vi "Single Tone Audio Measurements (N Ch).vi"(6 "units settings":T2, 8 "error in":errorcluster, 10 "measurement settings":T5={"Band start"=20.0, "Band stop"=20000.0, "Amplitude"=1.0, "Frequency"=1000.0, "Full scale range"=3.16}, 11 "waveforms":waveform(dbl)[](array[waveform])) -> (0 "error out":errorcluster, 1 "spectra":cluster{"x0":dbl, "dx":dbl, "magnitude":dbl[]}[](array[cluster]), 2 "waveforms":waveform(dbl)[](array[waveform]), 3 "results":T1[](array[typedef]))   [LabVIEW 2021]
uses:
  controls/single tone audio measurement settings.ctl
  controls/units settings.ctl
  controls/units - snr.ctl
  controls/units - ratio.ctl
  controls/single tone audio measurements.ctl
  <vilib>/addons/_NISVFA/_Shared subVIs/Common/SVL Set dB Reference (N Ch - 1 Ref).vi
  <vilib>/addons/Sound and Vibration/svt_Single Tone Measurements/SVT Spurious Free Dynamic Range (Frequency) (1 Ch).vi
  <vilib>/addons/_NISVFA/_Spectrum Processing/SVFA Unit Conversion (Complex) (1 Ch).vi
  <vilib>/addons/_NISVFA/_Shared subVIs/Common/SVL Set dB Reference (1 Ch).vi
  <vilib>/addons/_NISVFA/_Spectrum Processing/SVFA Get Spectrum Subset.vi
  <vilib>/addons/_NISVFA/_Spectrum Processing/SVFA Get Spectrum Subset (Complex) (1 Ch).vi
  <vilib>/addons/_NISVFA/_Shared subVIs/Common/svc_Window Parameters.vi
  <vilib>/addons/_NISVFA/_Shared subVIs/Common/svc_Extract Single Tone Information (complex).vi
  <vilib>/addons/_NISVFA/_Shared subVIs/Common/svc_Check Frequency Range in Spectrum.vi
  <vilib>/addons/_NISVFA/_Spectrum Processing/SVFA Spectrum Peak Search.vi
  <vilib>/addons/_NISVFA/_Spectrum Processing/SVFA Spectrum Peak Search (1 Ch).vi
  <vilib>/addons/_NISVFA/_Shared subVIs/Common/svc_Spectrum Units.vi
  <vilib>/addons/_NISVFA/_Shared subVIs/Common/svc_Log View for Spectrum (1Ch).vi
  <vilib>/addons/_NISVFA/_Spectrum Processing/SVFA Unit Conversion (1 Ch).vi
  <vilib>/addons/_NISVFA/_Shared subVIs/Common/svc_Complex Datatype Defaults.vi
  <vilib>/addons/_NISVFA/_Shared subVIs/Common/SVL Set dB Reference (variant).vi
  <vilib>/addons/_NISVFA/_Shared subVIs/Common/svc_Build Unit Label for Frequency Range.vi
  <vilib>/addons/_NISVFA/_Spectrum Processing/SVFA Get Tone Amplitude and Phase (1 Ch).vi
  <vilib>/addons/_NISVFA/_Spectrum Processing/subVIs/svfa_Compute Complex Spectrum for Export.vi
  <vilib>/addons/_NISVFA/_Shared subVIs/Common/svc_Check Frequency Range in Bandwidth.vi
  <vilib>/addons/_NISVFA/_Shared subVIs/Common/svc_Convert Start and Stop to Start Index and Length.vi
  <vilib>/addons/_NISVFA/_Spectrum Processing/subVIs/svfa_Spectrum Peak Search.vi
  <vilib>/addons/_NISVFA/_Shared subVIs/Common/svc_Format Value (DBL).vi
  <vilib>/addons/_NISVFA/_Shared subVIs/Common/svc_Get Weighting Enum and Labels.vi
  <vilib>/addons/_NISVFA/_Shared subVIs/Common/svc_Engineering Units to Unit Label.vi
  <vilib>/addons/_NISVFA/_Shared subVIs/Common/svc_Surround NonAlpha String with Parentheses.vi
  <vilib>/dlg_ctls.llb/Space Constant.vi
  <vilib>/addons/_NISVFA/_Shared subVIs/Common/svc_Unwrap Phase.vi
  <vilib>/addons/_NISVFA/_Shared subVIs/Common/svc_Convert Spectrum Array to dB.vi
  <vilib>/addons/_NISVFA/_Spectrum Processing/subVIs/svfa_Conversion Utility (spectrum info).vi
  <vilib>/addons/_NISVFA/_Spectrum Processing/subVIs/svfa_Window Frequency Response.vi
  <vilib>/addons/_NISVFA/_Spectrum Processing/subVIs/svfa_Window Frequency Response (double array).vi
  <vilib>/Analysis/baseanly.llb/Dot Product.vi
  <vilib>/Analysis/baseanly.llb/Complex Dot Product.vi
  <vilib>/addons/_NISVFA/_Spectrum Processing/subVIs/svfa_Peak Rough Search Indices.vi
  <vilib>/addons/_NISVFA/_Shared subVIs/Common/svc_Unit Label Lexical Class.vi
  <vilib>/addons/_NISVFA/_Spectrum Processing/subVIs/svfa_Peak to RMS to Peak2Peak.vi
  <vilib>/addons/_NISVFA/_Spectrum Processing/subVIs/svfa_Mag to Mag2.vi
  <vilib>/addons/_NISVFA/_Spectrum Processing/subVIs/svfa_Linear to dB.vi
  <vilib>/addons/_NISVFA/_Spectrum Processing/subVIs/svfa_dBrefA to dBrefB.vi
  <vilib>/addons/_NISVFA/_Spectrum Processing/subVIs/svfa_Spectrum to Spectral Density.vi
  <vilib>/addons/_NISVFA/_Spectrum Processing/subVIs/svfa_Rect Window Frequency Response.vi
  <vilib>/addons/_NISVFA/_Spectrum Processing/subVIs/svfa_Cosine Window Coefficients.vi
  <vilib>/addons/_NISVFA/_Shared subVIs/Common/svc_Caller VI Returned in Error Source.vi
  <vilib>/addons/Sound and Vibration/svt_Single Tone Measurements/SVT Gain (Time) (1 Ch).vi
  <vilib>/addons/Sound and Vibration/svt_Distortion/SVT SNR without Harmonics (Frequency) (1 Ch).vi
  <vilib>/addons/_NISVFA/_Spectrum Processing/SVFA Extract Single Tone Information (Complex) (1 Ch).vi
  <vilib>/addons/Sound and Vibration/svt_Single Tone Measurements/SVT Dynamic Range (Frequency) (1 Ch).vi
  <vilib>/addons/Sound and Vibration/svt_Distortion/subVIs/sv_Check Data Valid (Audio) (1 Ch).vi
  <vilib>/addons/_NISVFA/_Shared subVIs/Common/svc_Convert Frequency to Frequency String.vi
  <vilib>/Analysis/4window.llb/window parameters.vi
  <vilib>/Analysis/4window.llb/Window Properties.vi
  <vilib>/Analysis/4window.llb/Window Properties by Name.vi
  <vilib>/addons/_NISVFA/_Spectrum Processing/subVIs/svfa_Spectrum Peak Tone Search and Estimation (complex).vi
  <vilib>/measure/masignal.llb/Tones and Noise Waveform.vi
  <vilib>/addons/_NISVFA/_Shared subVIs/Common/svc_FFT with Window.vi
  <vilib>/Analysis/1siggen.llb/Square Wave.vi
  <vilib>/addons/_NISVFA/_Spectrum Processing/subVIs/svfa_Three Finger Peak Search.vi
  <vilib>/addons/Sound and Vibration/svt_Distortion/subVIs/sv_Peak View Amplitude (1 Ch).vi
  <vilib>/addons/Sound and Vibration/svt_Single Tone Measurements/SoundVib_SingleTone.lvlib
  <vilib>/addons/Sound and Vibration/svt_Distortion/SoundVib_Distortion.lvlib
  controls/audio controls.lvlib
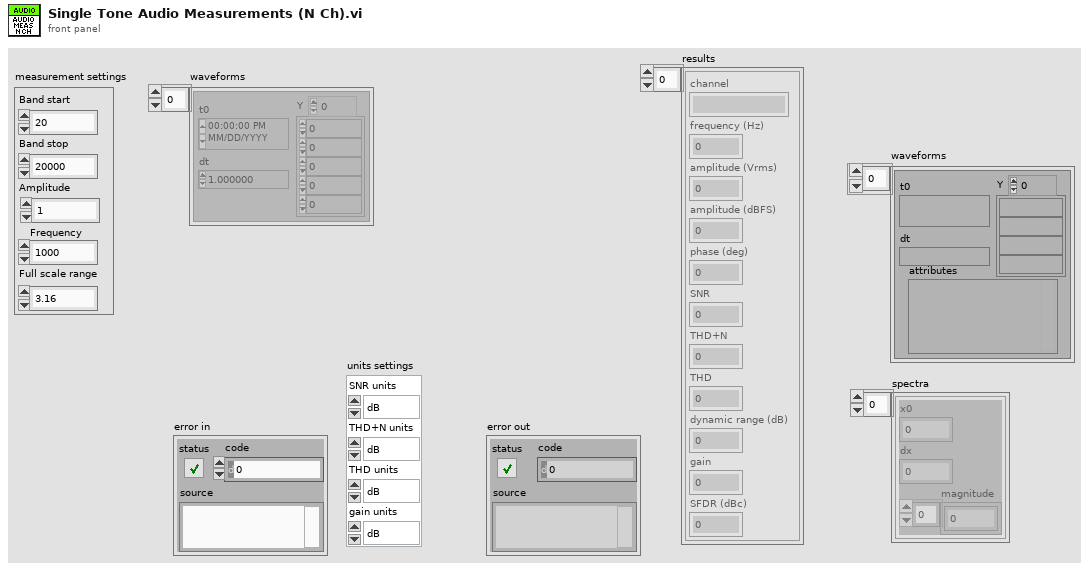
[diagram p1: front panel]
types:
  T1 = typedef "audio controls.lvlib/single tone audio measurements.ctl" = cluster{"channel":string, "frequency (Hz)":dbl, "amplitude (Vrms)":dbl, "amplitude (dBFS)":dbl, "phase (deg)":dbl, "SNR":dbl, "THD+N":dbl, "THD":dbl, "dynamic range (dB)":dbl, "gain":dbl, "SFDR (dBc)":dbl}
  T2 = typedef "audio controls.lvlib/units settings.ctl" = cluster{"SNR units":T3, "THD+N units":T4, "THD units":T4, "gain units":T4}
  T3 = typedef "audio controls.lvlib/units - snr.ctl" = enum32{"dB", "x/y"}
  T4 = typedef "audio controls.lvlib/units - ratio.ctl" = enum32{"dB", "%", "x/y"}
  T5 = typedef "single tone audio measurement settings.ctl" = cluster{"Band start":dbl, "Band stop":dbl, "Amplitude":dbl, "Frequency":dbl, "Full scale range":dbl}
  T6 = cluster{"start frequency":dbl, "stop frequency":dbl}
  T7 = cluster{"SNR units":enum16{"dB", "linear ratio", "%"}, "detected fundamental amplitude units":enum16{"EU rms", "EU peak", "EU peak-peak"}}
  T8 = cluster{"gain units":enum16{"dB", "linear ratio"}, "detected fundamental amplitude units":enum16{"EU rms", "EU peak", "EU peak-peak"}}
  T9 = enum16{"no change", "spectrum", "spectral density"}
  T10 = cluster{"linear/dB":enum16{"no change", "linear", "dB"}, "dB reference (0: no change)":dbl, "power/magnitude":enum16{"no change", "power", "magnitude"}, "view":enum16{"no change", "rms", "peak", "peak-peak"}}
  T11 = typedef "svc_Spectrum Info.ctl" = cluster{"channel name":string, "description":string, "x-axis units":T12, "spectral info":cluster{"spectrum type":T13, "linear/dB":enum16{"linear", "dB"}, "window":u16, "window size":i32, "FFT size":i32}, "engineering units":T14, "custom label":string, "dB reference [EU]":dbl, "peak units":enum16{"rms", "peak", "peak-peak"}, "weighting filter":T15, "spectral density?":bool, "unit label":string, "spectrum skewed?":bool, "complimentary spectrum units":T16}
  T12 = typedef "svc_X-Axis Units.ctl" = u16
  T13 = typedef "svc_Spectrum Type.ctl" = enum16{"FFT Spectrum [complex]", "Amplitude [Magnitude]", "Power [Magnitude^2]", "Cross Spectrum [complex]", "Frequency Response [Complex]"}
  T14 = typedef "svc_Engineering Units Text Ring.ctl" = u16
  T15 = typedef "svc_Weighting Filter Text Ring.ctl" = u16
  T16 = typedef "svc_Complimentary Spectrum Units.ctl" = enum16{"none", "radians", "degrees", "cycles", "imaginary"}
  T17 = cluster{"complex spectrum response":cluster{"f0":dbl, "df":dbl, "complex spectrum":cdb[]}, "spectrum info":T11}
  T18 = cluster{"frequency [Hz]":dbl, "amplitude [EU pk]":dbl, "phase (deg)":dbl}
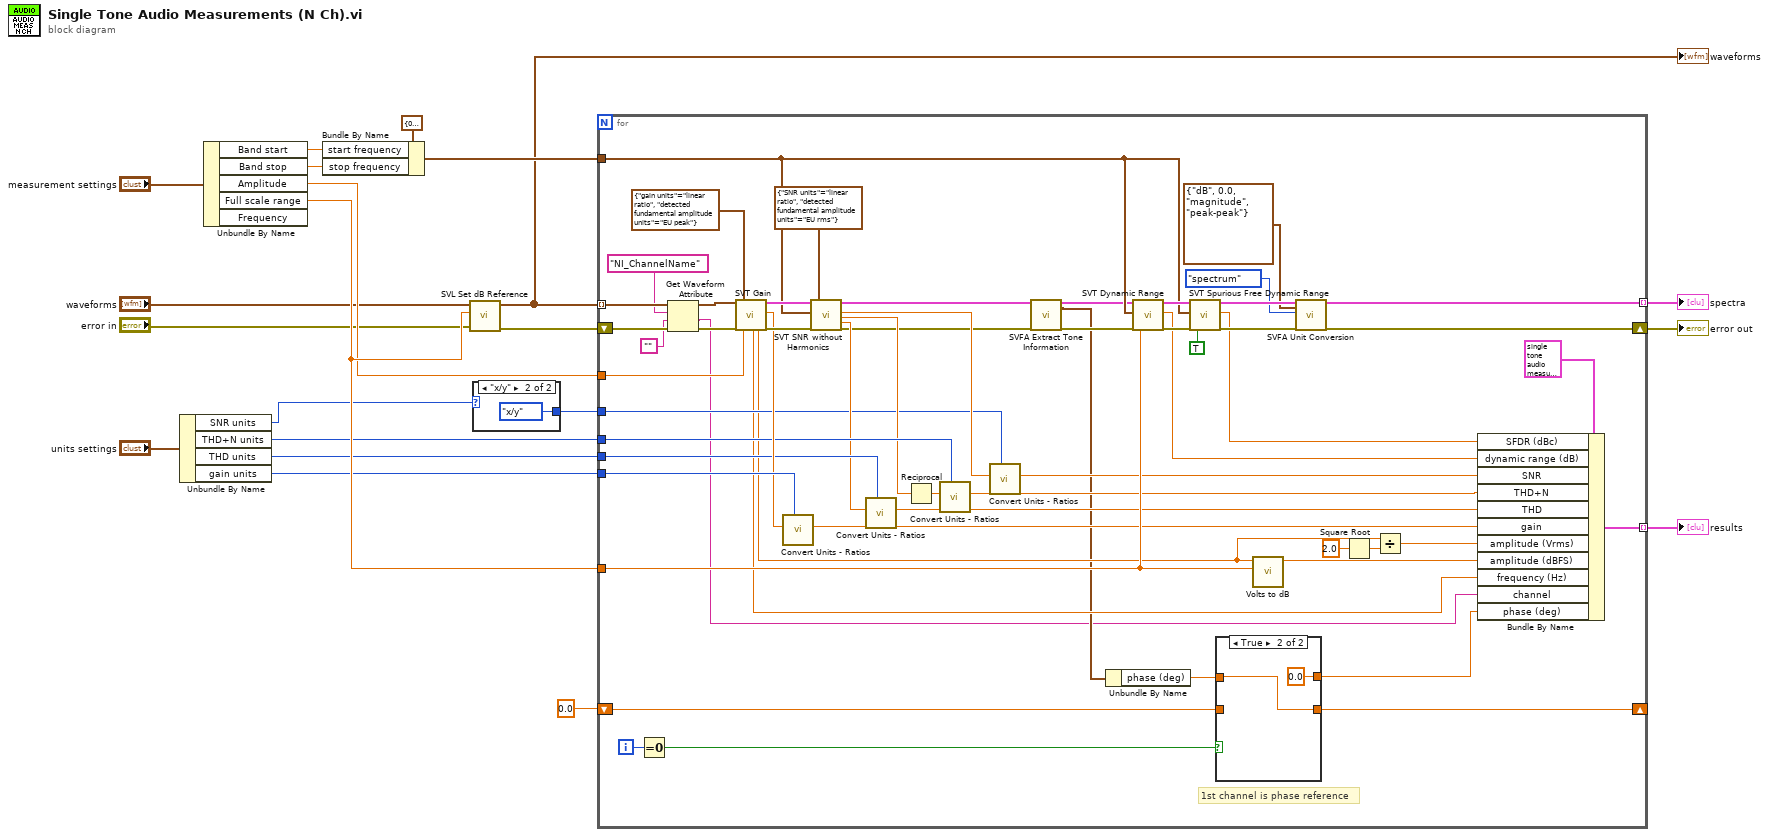
[diagram p0: block diagram]
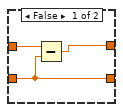
[diagram p2: hidden frame]
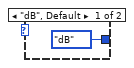
[diagram p3: hidden frame]
diagram:
  n1 = Unbundle By Name("units settings") -> ("SNR units"=w8:T3, "THD+N units"=w10:T4, "THD units"=w9:T4, "gain units"=w11:T4)
  n2 = Unbundle By Name("measurement settings") -> ("Band start"=w20:dbl, "Band stop"=w21:dbl, "Amplitude"=w14:dbl, "Full scale range"=w16:dbl)  [unwired: 1 out]
  n3 = Bundle By Name(cluster=T6 {"start frequency"=0.0, "stop frequency"=0.0} ("frequency range"), "start frequency"=w20, "stop frequency"=w21) -> (w18:T6)
  n4 = call-poly <vilib>:"SVL Set dB Reference.vi"("error in (no error)"="error in", "dB reference [EU]"=w16, "scaled signals in [EU]"="waveforms") -> ("error out"=w15:errorcluster, "scaled signals out [EU]"=w4:waveform(dbl)[])  [unwired: 7 in]
  "waveforms" <- w4
  n5 = case shown="\"x/y\"" w8 {
    tunnel: [units_-_ratio."dB" ("gain units") units_-_ratio."x/y" ("gain units")] -> w7
    frame "dB", Default {
    }
    frame "x/y" {
    }
  }
  n6 = for {
    tunnel: w18 -> [w69]
    tunnel: w16 -> [w68]
    tunnel: [w64] -> w2 mode=indexing
    tunnel: w14 -> [w63]
    tunnel: w11 -> [w62]
    tunnel: w10 -> [w59]
    tunnel: w9 -> [w53]
    tunnel: w7 -> [w50]
    tunnel: [w43] -> w1 mode=indexing
    shift-right: [w42] -> w5
    shift-left: w15 -> [w28]
    tunnel: w4 -> [w30] mode=indexing
    shift-right: [w32] -> _
    shift-left: 0.0 -> [w34]
    i -> [w36]
    # "1st channel is phase reference"
    n7 = Equal To 0?(x=w36) -> (x = 0?=w35:bool)
    n8 = Get Waveform Attribute(4:w28, 5:"", 6:"NI_ChannelName" ("name"), 7:w30) -> (0:w27:errorcluster, 1:w24:string, 3:w29:waveform(dbl))  [unwired: 1 out]
    n9 = call-poly <vilib>:"SVT Gain.vi"("scaled signal [EU]"=w29, "error in (no error)"=w27, "desired units"=T8 {"gain units"=enum."linear ratio", "detected fundamental amplitude units"=enum."EU peak"}, "amplitude [EU peak]"=w63) -> ("detected fundamental\nfrequency [Hz]"=w49:dbl, "detected fundamental\namplitude"=w44:dbl, "complex spectrum"=w74:T17, "gain"=w61:dbl, "error out"=w75:errorcluster)  [unwired: 10 in, 1 out]
    n10 = call "Convert Units - Ratios.vi"("gain units"=w62, "linear ratio"=w61) -> ("converted ratio"=w60:dbl)  [unwired: 9 in]
    n11 = call-poly <vilib>:"SVT SNR without Harmonics.vi"("complex spectrum"=w74, "frequency range"=w69, "error in (no error)"=w75, "desired units"=T7 {"SNR units"=enum."linear ratio", "detected fundamental amplitude units"=enum."EU rms"}) -> ("complex spectrum"=w41:T17, "SNR (without harmonics)"=w58:dbl, "SINAD"=w55:dbl, "THD"=w52:dbl, "error out"=w40:errorcluster)  [unwired: 8 in, 3 out]
    n12 = call "Convert Units - Ratios.vi"("gain units"=w53, "linear ratio"=w52) -> ("converted ratio"=w51:dbl)  [unwired: 9 in]
    n13 = Reciprocal(x=w55) -> (1/x=w56:dbl)
    n14 = call "Convert Units - Ratios.vi"("gain units"=w59, "linear ratio"=w56) -> ("converted ratio"=w54:dbl)  [unwired: 9 in]
    n15 = call "Convert Units - Ratios.vi"("gain units"=w50, "linear ratio"=w58) -> ("converted ratio"=w57:dbl)  [unwired: 9 in]
    n16 = call-poly <vilib>:"SVFA Extract Tone Information.vi"("complex spectrum"=w41, "error in"=w40) -> ("complex spectrum"=w39:T17, "detected tone"=w37:T18, "error out"=w38:errorcluster)  [unwired: 14 in, 1 out]
    n17 = Unbundle By Name(w37) -> ("phase (deg)"=w33:dbl)
    n18 = call-poly <vilib>:"SVT Dynamic Range.vi"("complex spectrum"=w39, "frequency range"=w69, "error in (no error)"=w38, "full scale amplitude [EU peak]"=w68) -> ("dup complex spectrum"=w78:T17, "dynamic range"=w66:dbl, "error out"=w79:errorcluster)  [unwired: 10 in, 3 out]
    n19 = call-poly <vilib>:"SVT Spurious Free Dynamic Range.vi"("complex spectrum"=w78, "frequency range"=w69, "error in (no error)"=w79, "exclude harmonics"=TRUE) -> ("complex spectrum"=w72:T17, "spurious free dynamic range"=w67:dbl, "error out"=w73:errorcluster)  [unwired: 8 in, 5 out]
    n20 = case shown="True" w35 {
      tunnel: w34 -> [w82 _]
      tunnel: w33 -> [w83 w85]
      tunnel: [w81 0.0] -> w31
      tunnel: [w82 w85] -> w32
      frame False {
        n21 = Subtract(x=w83, y=w82) -> (x-y=w81:dbl)
      }
      frame True {
      }
    }
    n22 = call "Volts to dB.vi"("Full scale range"=w68, "Voltage(V)"=w44) -> ("Voltage(dB)"=w48:dbl)  [unwired: 9 in]
    n23 = call-poly <vilib>:"SVFA Unit Conversion.vi"("complex spectrum"=w72, "desired scaling"=T10 {"linear/dB"=enum."dB", "dB reference (0: no change)"=0.0, "power/magnitude"=enum."magnitude", "view"=enum."peak-peak"}, "spectral density desired"=T9."spectrum", "error in (no error)"=w73) -> ("converted spectrum"=w43:cluster{"x0":dbl, "dx":dbl, "magnitude":dbl[]}, "error out"=w42:errorcluster)  [unwired: 10 in, 4 out]
    n24 = Square Root(x=2.0 ("y")) -> (sqrt(x)=w47:dbl)
    n25 = Divide(x=w44, y=w47) -> (x/y=w45:dbl)
    n26 = Bundle By Name(cluster=T1 {"channel"="", "frequency (Hz)"=0.0, "amplitude (Vrms)"=0.0, "amplitude (dBFS)"=0.0, "phase (deg)"=0.0, "SNR"=0.0, "THD+N"=0.0, "THD"=0.0, "dynamic range (dB)"=0.0, "gain"=0.0, "SFDR (dBc)"=0.0} ("results"), "SFDR (dBc)"=w67, "dynamic range (dB)"=w66, "SNR"=w57, "THD+N"=w54, "THD"=w51, "gain"=w60, "amplitude (Vrms)"=w45, "amplitude (dBFS)"=w48, "frequency (Hz)"=w49, "channel"=w24, "phase (deg)"=w31) -> (w64:T1)
  }
  "error out" <- w5
  "results" <- w2
  "spectra" <- w1
